vi "Start Daemon.vi"(8 "error in (no error)":errorcluster, 11 "WAMP Client in":refnum<class "WAMP Client.lvclass">) -> (0 "error out":errorcluster, 3 "WAMP Client out":refnum<class "WAMP Client.lvclass">)   [LabVIEW 2020, in "wamplv.lvlib" / "WAMP Client.lvclass"]
uses:
  WAMP Client.lvclass
  Daemon.vi
  WAMP Client.lvclass/WAMP Client.ctl
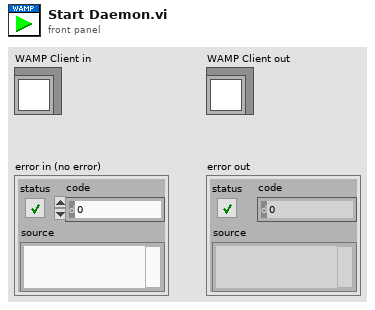
[diagram p1: front panel]
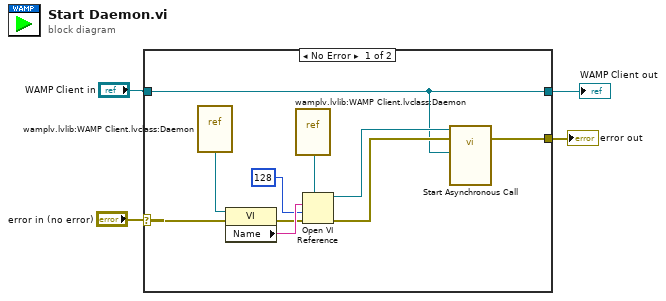
[diagram p0: block diagram]
diagram:
  n1 = case shown="No Error" "error in (no error)" {
    selector: "error in (no error)" -> [w7 w15]
    tunnel: [w10 w15] -> w1
    tunnel: "WAMP Client in" -> [w5 w16]
    tunnel: [w5 w16] -> w2
    frame No Error {
      n2 = vi-ref "wamplv.lvlib:WAMP Client.lvclass:Daemon.vi"() -> (w13:refnum<vi>)
      n3 = property class="VI"(reference=w13, error in=w7) -> (error out=w8:errorcluster, "Name"=w11:string)  [unwired: 1 out]
      n4 = vi-ref "wamplv.lvlib:WAMP Client.lvclass:Daemon.vi"() -> (w12:refnum<vi>)
      n5 = Open VI Reference(type specifier VI Refnum (for type only)=w12, vi path=w11, options=128, error in (no error)=w8) -> (vi reference=w14:refnum<vi>, error out=w6:errorcluster)  [unwired: 2 in]
      n6 = call-by-ref "Start Asynchronous Call"(reference=w14, error in=w6, "WAMP Client in"=w5) -> (error out=w10:errorcluster)  [unwired: 10 in, 2 out]
    }
    frame Error {
    }
  }
  "WAMP Client out" <- w2
  "error out" <- w1
